vi "BB_Siren_Run.vi"(6 "Low Freq in":dbl=440.0, 8 "Error In":errorcluster, 9 "sampling info":cluster{"Fs":dbl, "#s":dbl}, 10 "Active":bool, 11 "Task ID In":T1 format="%.0x") -> (0 "error out":errorcluster, 3 "task ID out":T1 format="%.0x")   [LabVIEW 2012]
uses:
  <vilib>/sound2/lvsound2.llb/Sound Output Task ID.ctl
  <vilib>/sound2/lvsound2.llb/Sound Output Set Volume (Single).vi
  <vilib>/sound2/lvsound2.llb/Sound Output Write (DBL Single).vi
  <vilib>/measure/NI_MABase.lvlib
panel:
  in  "High Freq in":dbl=1480.0
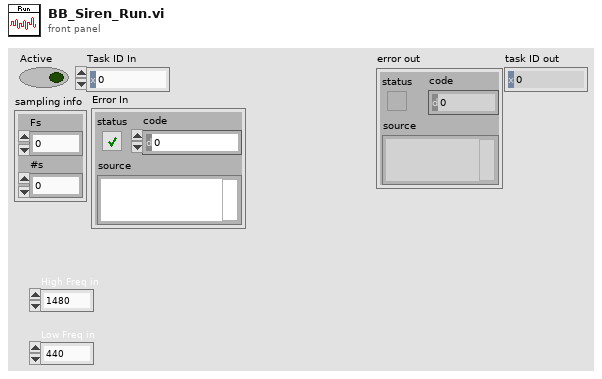
[diagram p1: front panel]
types:
  T1 = typedef "Sound Output Task ID.ctl" = u32
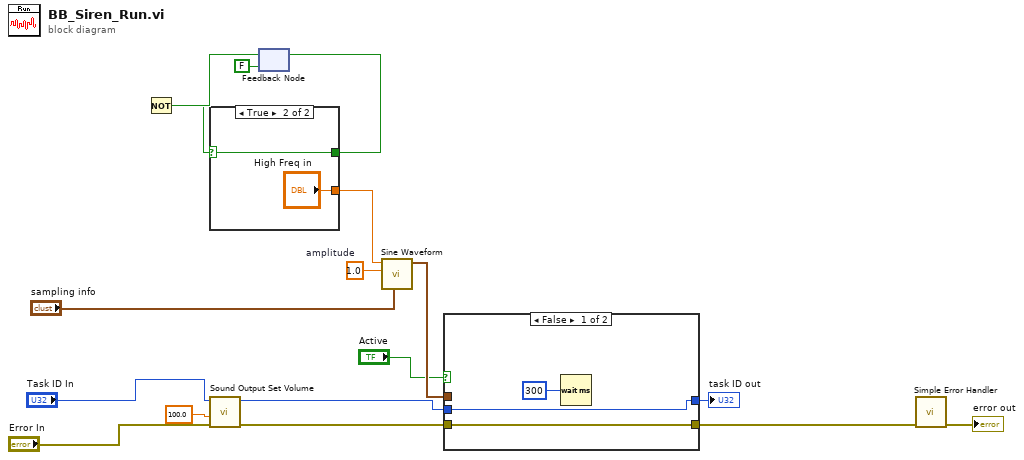
[diagram p0: block diagram]
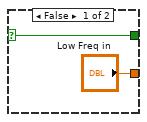
[diagram p2: hidden frame]
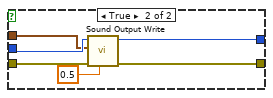
[diagram p3: hidden frame]
diagram:
  w12 = 1.0  # amplitude
  n1 = call-poly <vilib>:"Sound Output Set Volume.vi"("error in (no error)"="Error In", "volume"=100.0 ("Volume"), "task ID"="Task ID In") -> ("error out"=w11:errorcluster, "task ID out"=w10:T1)  [unwired: 7 in]
  n2 = feedback #1(FALSE) -> (w6:bool)
  n3 = Not(x=w6) -> (.not. x?=w1:bool)
  n4 = case shown="True" w1 {
    selector: w1 -> [w18 w20]
    tunnel: ["Low Freq in" "High Freq in"] -> w13
    tunnel: [w18 w20] -> w5
    frame False {
    }
    frame True {
    }
  }
  n5 = feedback-in #1(w5) -> ()
  n6 = call <vilib>:"Sine Waveform.vi"("sampling info"="sampling info", "amplitude"=w12, "frequency"=w13) -> ("signal out"=w8:waveform(dbl))  [unwired: 7 in, 1 out]
  n7 = case shown="False" "Active" {
    tunnel: [w23 w30] -> w2
    tunnel: [w22 w29] -> w3
    tunnel: w11 -> [w22 w28]
    tunnel: w10 -> [w23 w27]
    tunnel: w8 -> [_ w26]
    frame False {
      n8 = Wait (ms)(milliseconds to wait=u32 300) -> ()  [unwired: 1 out]
    }
    frame True {
      n9 = call-poly <vilib>:"Sound Output Write.vi"("timeout (sec)"=0.5, "error in (no error)"=w28, "data"=w26, "task ID"=w27) -> ("error out"=w29:errorcluster, "task ID out"=w30:T1)  [unwired: 6 in]
    }
  }
  "task ID out" <- w2
  n10 = call <vilib>:"Simple Error Handler.vi"("error in (no error)"=w3) -> ("error out"=→"error out":errorcluster)  [unwired: 4 in, 4 out]
